vi "View-Palette.vi"(11 "Array":refnum<class "Material-Palette.lvclass">[](array[class])) -> ()   [LabVIEW 2021, in "TSC Material Theme.lvlib" / "Material-Palette.lvclass"]
doc: "read material palette data\n\n<b>Code Developed By:</b>\nTechnology Service Corporation\nwww.tsc.com/atcs\n\nDeveloper:\nDaniel Coons"
uses:
  Material-Palette.lvclass
  Material-Palette.lvclass/Material-Palette.ctl
panel:
  out "palettes":T1(array[cluster])
  # "Primary"
  # "Secondary"
  # "Tertiary"
  # "Neutral"
  # "Neutral-Variant"
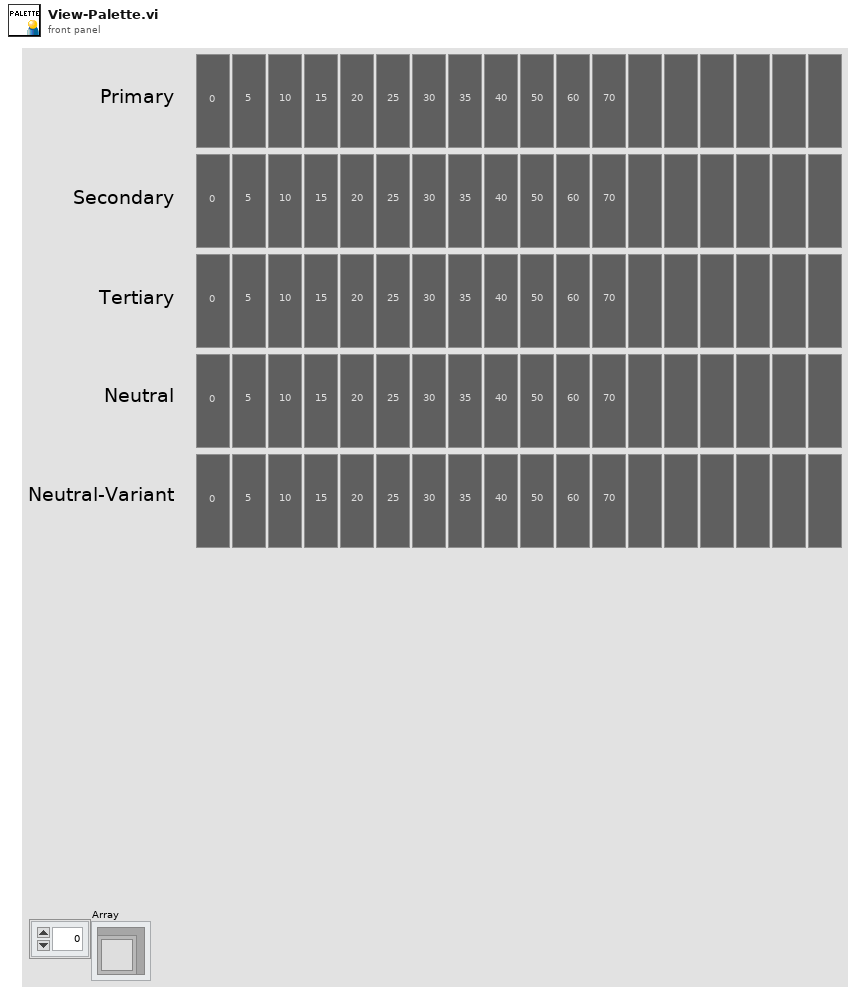
[diagram p1: front panel]
types:
  T1 = cluster{"0":u32, "5":u32, "10":u32, "15":u32, "20":u32, "25":u32, "30":u32, "35":u32, "40":u32, "50":u32, "60":u32, "70":u32, "80":u32, "90":u32, "95":u32, "98":u32, "99":u32, "100":u32}[]
  T2 = cluster{"0":u32, "5":u32, "10":u32, "15":u32, "20":u32, "25":u32, "30":u32, "35":u32, "40":u32, "50":u32, "60":u32, "70":u32, "80":u32, "90":u32, "95":u32, "98":u32, "99":u32, "100":u32}
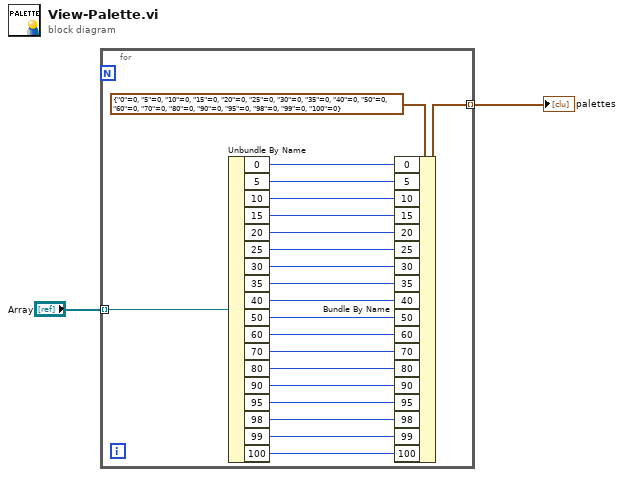
[diagram p0: block diagram]
diagram:
  n1 = for {
    tunnel: "Array" -> [w23] mode=indexing
    tunnel: [w3] -> w1 mode=indexing
    n2 = Unbundle By Name(w23) -> ("0"=w22:u32, "5"=w20:u32, "10"=w19:u32, "15"=w18:u32, "20"=w17:u32, "25"=w16:u32, "30"=w15:u32, "35"=w14:u32, "40"=w13:u32, "50"=w12:u32, "60"=w11:u32, "70"=w10:u32, "80"=w9:u32, "90"=w8:u32, "95"=w7:u32, "98"=w6:u32, "99"=w5:u32, "100"=w4:u32)
    n3 = Bundle By Name(cluster=T2 {"0"=0, "5"=0, "10"=0, "15"=0, "20"=0, "25"=0, "30"=0, "35"=0, "40"=0, "50"=0, "60"=0, "70"=0, "80"=0, "90"=0, "95"=0, "98"=0, "99"=0, "100"=0} ("Tone"), "0"=w22, "5"=w20, "10"=w19, "15"=w18, "20"=w17, "25"=w16, "30"=w15, "35"=w14, "40"=w13, "50"=w12, "60"=w11, "70"=w10, "80"=w9, "90"=w8, "95"=w7, "98"=w6, "99"=w5, "100"=w4) -> (w3:T2)
  }
  "palettes" <- w1
